vi "Actor Core.vi"(8 "error in":errorcluster, 11 "Excel Saver in":refnum<class "Excel Saver.lvclass">) -> (0 "error out":errorcluster, 3 "Actor out":refnum<class "Actor.lvclass">)   [LabVIEW 2016, in "Data Saving.lvlib" / "Excel Saver.lvclass"]
doc: "(<B>Filename</B>: Actor Framework.lvlib:Actor.lvclass:Actor Core.vi)\n\nReceives messages to the actor, reacts to them, and initiates any error handling that may shut the actor down.\n\nDescendant classes may override this VI to append parallel tasks for the actor to complete while it handles messages. Overrides use the Call Parent Method node."
uses:
  Excel Saver.lvclass
  <vilib>/ActorFramework/Actor/Actor.lvclass
  Abstract Saver/Abstract Saver.lvclass
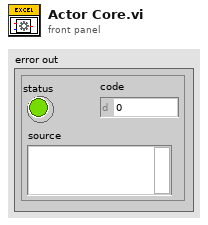
[diagram p1: front panel]
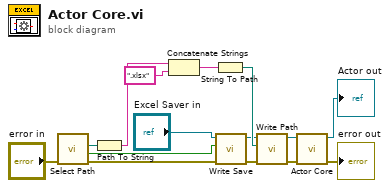
[diagram p0: block diagram]
diagram:
  n1 = call "Select Path.vi"("error in"="error in") -> ("error out"=w5:errorcluster, "Save?"=w1:bool, "selected path"=w7:path)  [unwired: 5 in, 1 out]
  n2 = Path To String(path=w7) -> (string=w8:string)
  n3 = Concatenate Strings(w8, ".xlsx" ("string")) -> (w9:string)
  n4 = String To Path(string=w9) -> (path=w6:path)
  n5 = call-dynamic "Write Save.vi"("error in (no error)"=w5, "Save"=w1, "Excel Saver in"="Excel Saver in") -> ("error out"=w2:errorcluster, "Excel Saver out"=w3:refnum<class "Excel Saver.lvclass">)  [unwired: 7 in]
  n6 = call-dynamic "Write Path.vi"("error in (no error)"=w2, "Path"=w6, "Abstract Saver in"=w3) -> ("error out"=w14:errorcluster, "Abstract Saver out"=w13:refnum<class "Excel Saver.lvclass">)  [unwired: 7 in]
  n7 = call-parent "Actor Core.vi"("error in"=w14, "Actor in"=w13) -> ("error out"=→"error out":errorcluster, "Actor out"=→"Actor out":refnum<class "Actor.lvclass">)  [unwired: 8 in]
